vi "Update Image List.vi"(8 "error in (no error)":errorcluster, 10 "Image Name":string, 11 "UserInterface in":refnum<class "UserInterface.lvclass">) -> (0 "error out":errorcluster, 3 "UserInterface out":refnum<class "UserInterface.lvclass">)   [LabVIEW 2022 SP3, in "UserInterface.lvlib" / "UserInterface.lvclass"]
uses:
  UserInterface.lvclass
  UserInterface.lvclass/UserInterface.ctl
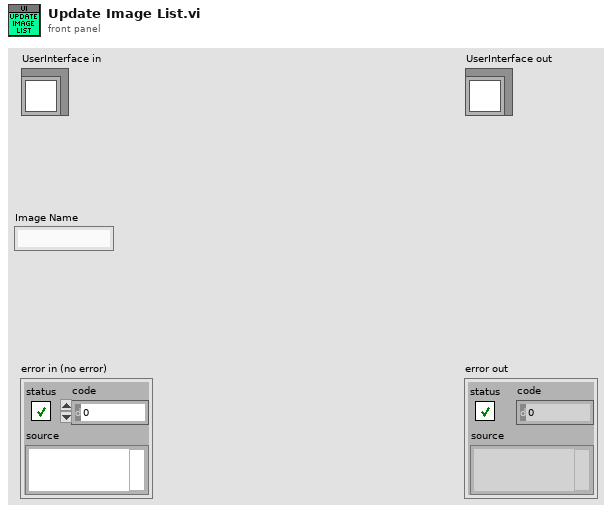
[diagram p1: front panel]
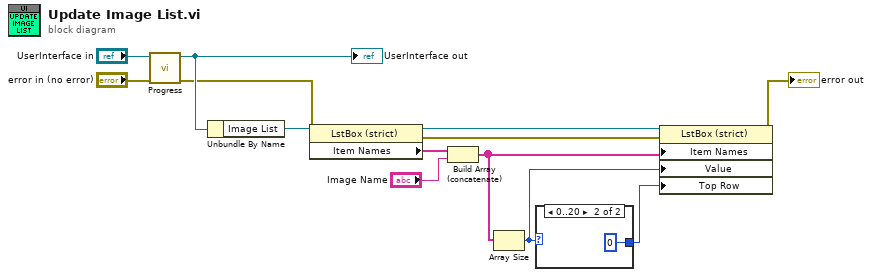
[diagram p0: block diagram]
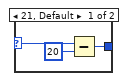
[diagram p2: hidden frame]
diagram:
  n1 = call "Progress.vi"("error in"="error in (no error)", "UserInterface in"="UserInterface in") -> ("error out"=w3:errorcluster, "UserInterface out"=w12:refnum<class "UserInterface.lvclass">)  [unwired: 8 in]
  "UserInterface out" <- w12
  n2 = Unbundle By Name(w12) -> ("Image List"=w10:refnum<vi>)
  n3 = property class="LstBox (strict)"(reference=w10, error in=w3) -> (reference out=w9:refnum<vi>, error out=w2:errorcluster, "Item Names"=w8:string[])
  n4 = Build Array (concatenate)(w8, "Image Name") -> (w7:string[])
  n5 = Array Size(array=w7) -> (size(s)=w5:i32)
  n6 = case shown="0..20" w5 {
    selector: w5 -> [w16 _]
    tunnel: [w14 0] -> w6
    frame 21, Default {
      n7 = Subtract(x=w16, y=20) -> (x-y=w14:i32)
    }
    frame 0..20 {
    }
  }
  n8 = property class="LstBox (strict)"(reference=w9, error in=w2, "Item Names"=w7, "Value"=w5, "Top Row"=w6) -> (error out=→"error out":errorcluster)  [unwired: 1 out]
